vi "NI6071E.GetDAQStatus.vi"(0 "i ref in":refnum<vi>, 4 "timeout ms (60000)":i32=60000, 5 "error in (no error)":errorcluster) -> (14 "i ref out":refnum<vi>, 16 "Status":string, 19 "error out":errorcluster)   [LabVIEW 2014, in "NI6071E.lvlib"]
uses:
  NI6071E.lvlib
  NI6071ECommandCluster.ctl
  NI6071ECommand.ctl
  lib.lib/DimLVEvent/LVDimInterface/LVDimInterface.lvlib
panel:
  in  "PPMA Command":T1=enum."ConfigureDAQ"
  in  "PPMA Command Cluster":T2
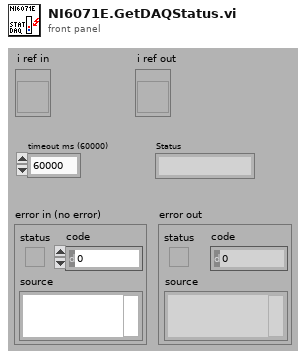
[diagram p1: front panel]
types:
  T1 = typedef "NI6071E.lvlib/NI6071ECommand.ctl" = enum16{"Ping", "Reset", "ConfigureDAQ", "StartDAQ", "StopDAQ", "GetDAQStatus", "ReadData", "SaveData", "CloseConnection"}
  T2 = typedef "NI6071E.lvlib/NI6071ECommandCluster.ctl" = cluster{"Command":string, "Data":string, "error out":errorcluster}
  T3 = typedef "NI6071E.lvlib/NI6071E.i attribute.ctl" = cluster{"NI6071E Server":string, "Port":u16, "NI6071E Config":T4, "NI6071E Start":T5, "Waveforms":waveform(dbl)[], "RT Error":errorcluster, "NI6071E Read":T6, "connection ID":refnum<k5>, "DAQ Status":string, "device (1)":i16, "DAQ Status Service ID":i32}
  T4 = typedef "NI6071E.lvlib/NI6071EConfig.ctl" = cluster{"device (1)":i16, "channels (0)":tag[], "buffer size (1000 scans)":i32, "[number of buffers] (1)":i32, "measurement mode structure":cluster{"measurement mode":u16, "reserved":u32}, "input limits (no change)":cluster{"high limit (0.0)":sgl, "low limit (0.0)":sgl}[], "coupling & input config (no change:0)":cluster{"coupling (no change:0)":enum16{"no change", "DC", "AC", "GND", "internal ref."}, "input config (no change:0)":u16}[]}
  T5 = typedef "NI6071E.lvlib/NI6071EStart.ctl" = cluster{"scan rate (40000 scans/sec)":sgl, "trigger type (analog)":enum16{"no trigger", "analog", "digital A", "digital A & B", "scan clock gate"}, "edge or slope \n(rising)":enum16{"no change", "rising", "falling"}, "number of buffers to acquire (1)":i32, "analog chan (PFI0) & level (2.00)":cluster{"trigger channel (empty)":string, "level (0.0)":sgl}, "[additional trig params]":cluster{"hysteresis (0.0)":sgl, "coupling (no change:0)":enum16{"no change", "DC", "AC"}, "delay (0 sec)":sgl, "skip count (0)":i32, "time limit (0 sec)":sgl}}
  T6 = typedef "NI6071E.lvlib/NI6071ERead.ctl" = cluster{"time limit in sec (-1:auto calculate)":sgl, "number of scans to read (-1:all)":i32}
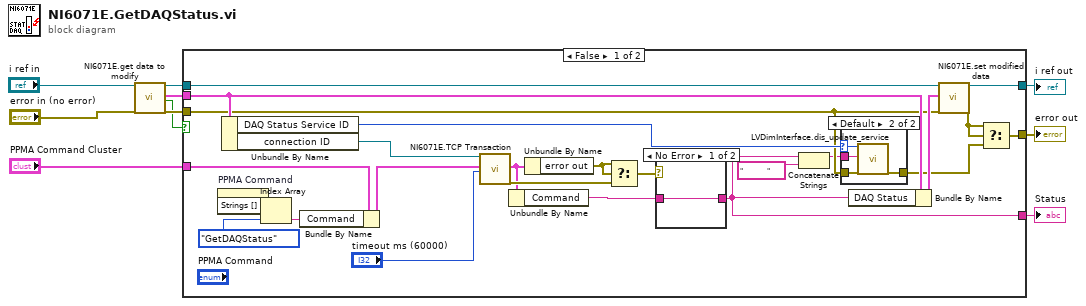
[diagram p0: block diagram]
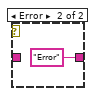
[diagram p2: hidden frame]
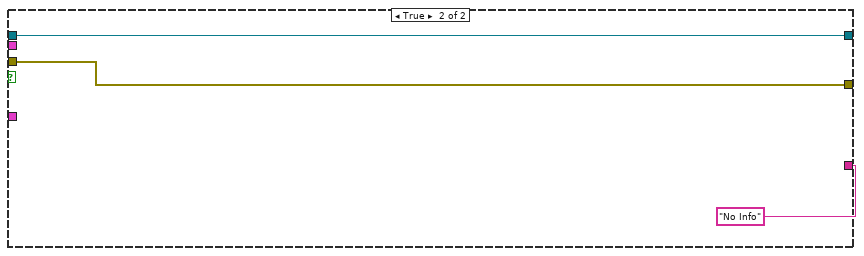
[diagram p4: hidden frame]
diagram:
  n1 = call "NI6071E.get data to modify.vi"("i ref in"="i ref in", "error in (no error)"="error in (no error)") -> ("i ref out"=w6:refnum<vi>, "i attribute"=w8:T3, "timed out"=w2:bool, "error out"=w7:errorcluster)  [unwired: 14 in]
  n2 = case shown="False" w2 {
    tunnel: w8 -> [w34 _]
    tunnel: w7 -> [w15 w43]
    tunnel: w6 -> [w33 w44]
    tunnel: [w32 w44] -> w5
    tunnel: [w30 w43] -> w4
    tunnel: "PPMA Command Cluster" -> [w27 _]
    tunnel: [w12 "No Info" ("Command")] -> w1
    frame False {
      n3 = property on="PPMA Command" class="Enum (strict)"() -> ("Strings []"=w25:string[])  [unwired: 2 in, 2 out]
      n4 = Unbundle By Name(w34) -> ("DAQ Status Service ID"=w17:i32, "connection ID"=w28:refnum<k5>)
      n5 = Index Array(array=w25, index=NI6071ECommand."GetDAQStatus" ("PPMA Command")) -> (element=w23:string)
      n6 = Bundle By Name(cluster=w27, "Command"=w23) -> (w26:T2)
      n7 = call "NI6071E.TCP Transaction.vi"("connection ID in"=w28, "NI6071E Command Cluster"=w26, "timeout ms (25000)"="timeout ms (60000)") -> ("NI6071E Response"=w19:T2, "error out"=w20:errorcluster)  [unwired: 14 in, 1 out]
      n8 = Unbundle By Name(w19) -> ("Command"=w14:string)
      n9 = Unbundle By Name(w19) -> ("error out"=w21:errorcluster)
      n10 = Select(t=w21, s=w21, f=w20) -> (s? t:f=w16:errorcluster)
      n11 = case shown="No Error" w16 {
        tunnel: [w35 "Error" ("Command")] -> w12
        tunnel: w14 -> [w35 _]
        frame No Error {
        }
        frame Error {
        }
      }
      n12 = Concatenate Strings(w12, "            " ("string")) -> (w13:string)
      n13 = case shown="Default" w17 {
        selector: w17 -> [_ w39]
        tunnel: w15 -> [w37 w41]
        tunnel: [w37 w40] -> w18
        tunnel: w13 -> [_ w38]
        frame -1 {
        }
        frame Default {
          n14 = call "LVDimInterface.dis_update_service.vi"("my_serviceID"=w39, "data"=w38, "error in (no error)"=w41) -> ("error out"=w40:errorcluster)  [unwired: 14 in, 2 out]
        }
      }
      n15 = Bundle By Name(cluster=w34, "DAQ Status"=w12) -> (w29:T3)
      n16 = call "NI6071E.set modified data.vi"("i ref in"=w33, "i attribute"=w29, "error in (no error)"=w15) -> ("i ref out"=w32:refnum<vi>, "error out"=w31:errorcluster)  [unwired: 15 in]
      n17 = Select(t=w31, s=w31, f=w18) -> (s? t:f=w30:errorcluster)
    }
    frame True {
    }
  }
  "i ref out" <- w5
  "error out" <- w4
  "Status" <- w1
